vi "计算文件间隔天数.vi"(10 "字符串":string) -> (3 "数值":dbl)   [LabVIEW 2014]
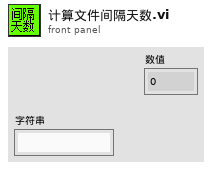
[diagram p1: front panel]
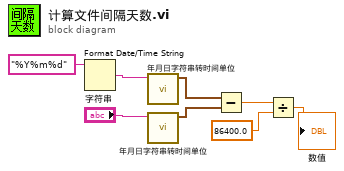
[diagram p0: block diagram]
diagram:
  n1 = Format Date/Time String(time format string (%c)="%Y%m%d") -> (date/time string=w1:string)  [unwired: 2 in]
  n2 = call "年月日字符串转时间单位.vi"("年月日字符串"=w1) -> ("time stamp"=w3:timestamp)  [unwired: 10 in]
  n3 = call "年月日字符串转时间单位.vi"("年月日字符串"="字符串") -> ("time stamp"=w8:timestamp)  [unwired: 10 in]
  n4 = Subtract(x=w3, y=w8) -> (x-y=w5:dbl)
  n5 = Divide(x=w5, y=86400.0) -> (x/y=→"数值":dbl)
